vi "Handle Error.vi"(8 "error in (no error)":errorcluster, 11 "VolatusCore in":refnum<class "VolatusCore.lvclass">) -> (0 "error out":errorcluster, 2 "stop actor?":bool=TRUE, 3 "VolatusCore out":refnum<class "VolatusCore.lvclass">)   [LabVIEW 2020, in "Volatus.lvlib" / "VolatusCore.lvclass"]
doc: "(<B>Filename</B>: Actor Framework.lvlib:Actor.lvclass:Handle Error.vi)\n\nDefines how the actor handles an error that occurred while processing a message. By default, this method does nothing except stop the actor."
uses:
  VolatusCore.lvclass
  VolatusCore.lvclass/VolatusCore.ctl
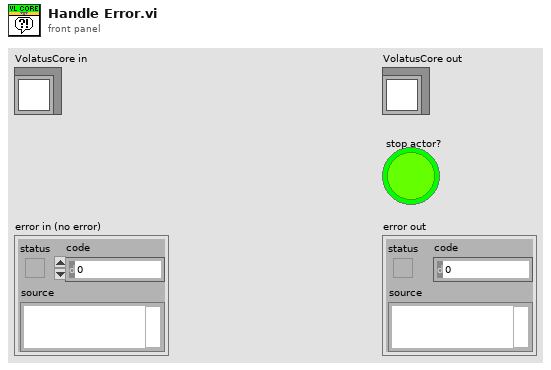
[diagram p1: front panel]
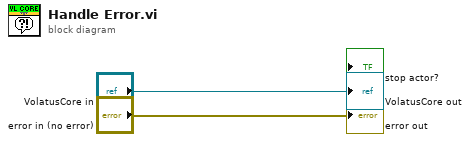
[diagram p0: block diagram]
diagram:
  "VolatusCore out" <- "VolatusCore in"
  "error out" <- "error in (no error)"
